vi "DSC TSV PRE-Process Files with Queues.vi"() -> ()   [LabVIEW 2019, in "LV-Data.PGSQL.lvclass"]
uses:
  LV-Data.PGSQL.lvclass
  <userlib>/_OpenG.lib/file/file.llb/Build Path - File Names Array__ogtk.vi
panel:
  out "appended path":path
  out "read loop":i32
  in  "Stop":bool
  out "conversion loop":i32
  in  "Folders":path
  in  "Number of row to read \nat a time":i32=10000
  in  "error in":errorcluster
  out "error out":errorcluster
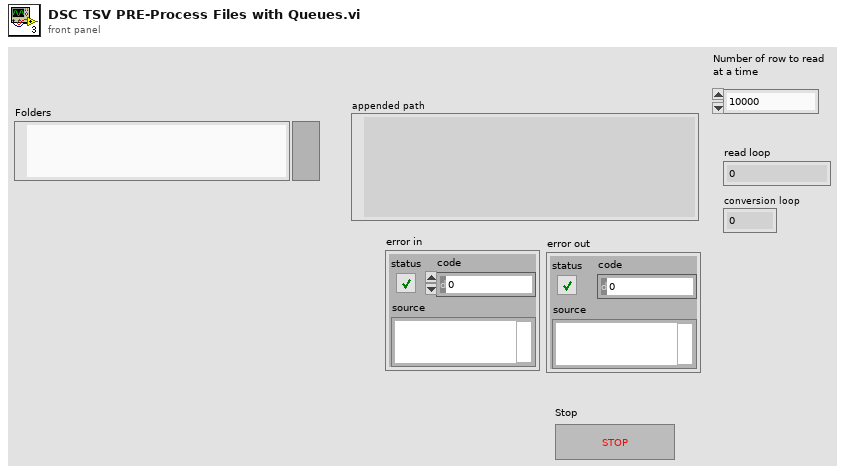
[diagram p1: front panel]
types:
  T1 = enum16{"open", "replace", "create", "open or create", "replace or create", "replace or create with confirmation"}
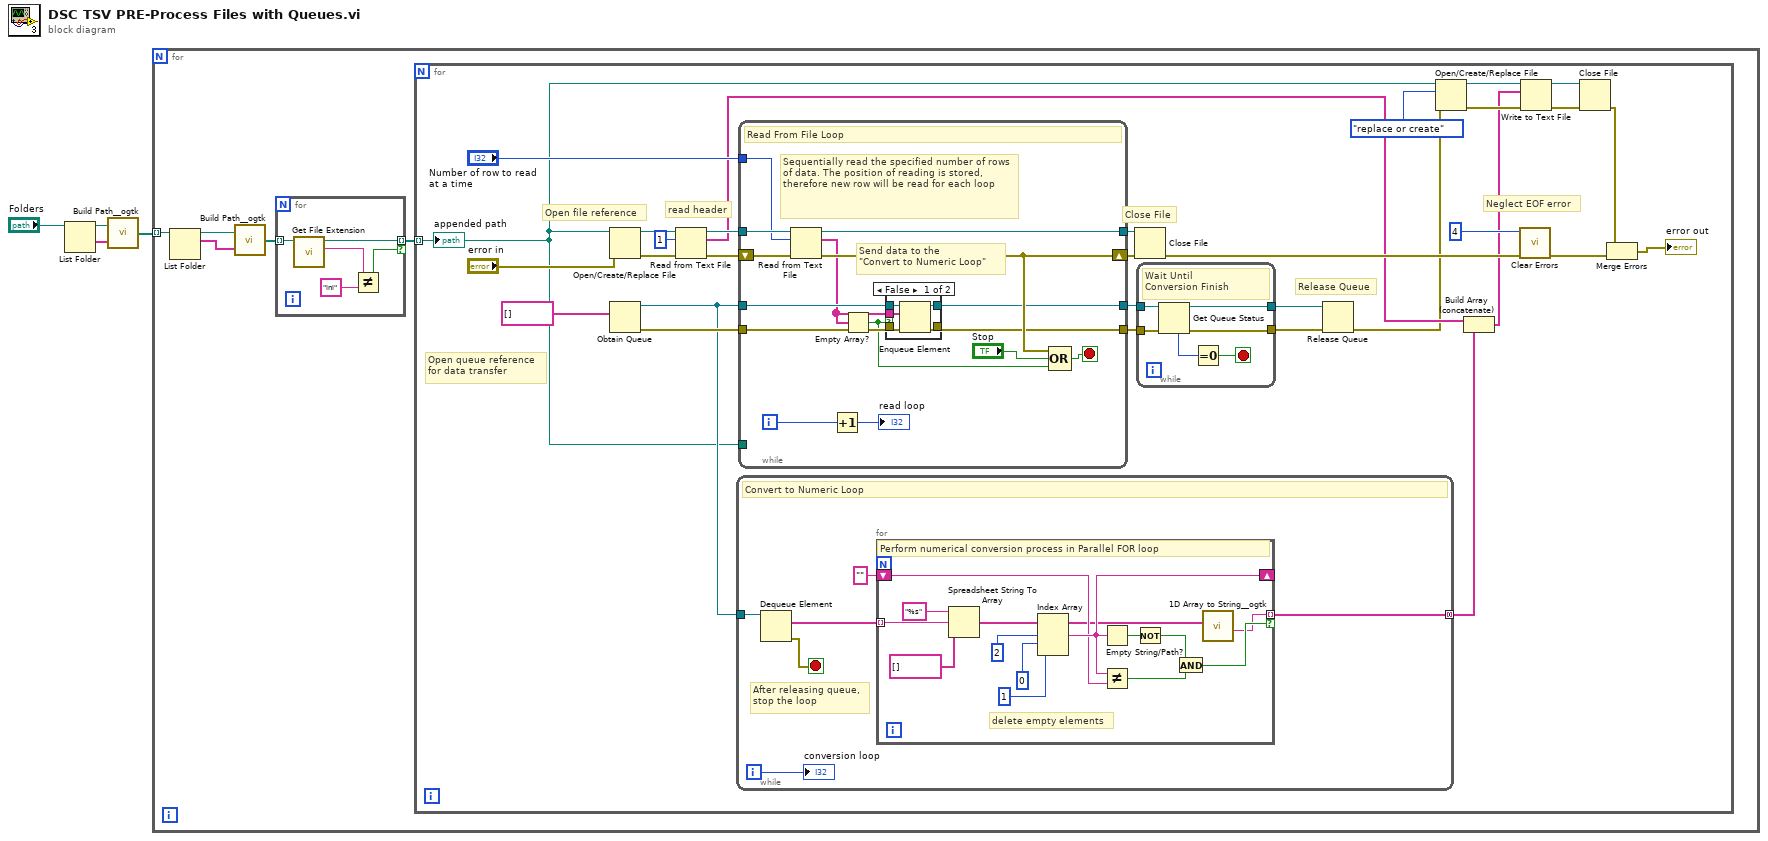
[diagram p0: block diagram]
diagram:
  n1 = List Folder(path="Folders") -> (path out=w3:path, folder names=w4:string[])  [unwired: 3 in, 2 out]
  n2 = call-poly <userlib>:"Build Path__ogtk.vi"("name or relative path"=w4, "base path"=w3) -> ("appended path"=w2:path[])
  n3 = for {
    tunnel: w2 -> [w9] mode=indexing
    n4 = List Folder(path=w9) -> (path out=w8:path, filenames=w7:string[])  [unwired: 3 in, 2 out]
    n5 = call-poly <userlib>:"Build Path__ogtk.vi"("name or relative path"=w7, "base path"=w8) -> ("appended path"=w6:path[])
    n6 = for {
      tunnel: w6 -> [w14] mode=indexing
      tunnel: [w13] -> w5 mode=indexing if=w10
      n7 = call <vilib>:"Get File Extension.vi"("file"=w14) -> ("lowercase file extension"=w12:string, "dup file"=w13:path)  [unwired: 6 in, 3 out]
      n8 = Not Equal?(x=w12, y="ini") -> (x != y?=w10:bool)
    }
    n9 = for {
      tunnel: w5 -> [w17] mode=indexing
      # "read header"
      # "Neglect EOF error"
      # "Release Queue"
      # "Close File"
      # "Open queue reference\nfor data transfer"
      # "Open file reference"
      n10 = Open/Create/Replace File(file path (use dialog)=w17, error in="error in") -> (refnum out=w34:refnum<file>, error out=w31:errorcluster)  [unwired: 4 in, 1 out]
      n11 = Obtain Queue(element data type=string[] [] ("形式文字列")) -> (queue out=w39:refnum<queue>, error out=w40:errorcluster)  [unwired: 4 in, 1 out]
      n12 = Read from Text File(file (use dialog)=w34, count=1, error in=w31) -> (refnum out=w33:refnum<file>, text=w23:string[], error out=w32:errorcluster)  [unwired: 1 in, 1 out]
      n13 = while {
        tunnel: w39 -> [w51]
        tunnel: [w46] -> w25 mode=concatenating
        i -> [w49]
        stop <- w50 stop-if-true
        # "After releasing queue,\nstop the loop"
        # "Convert to Numeric Loop"
        n14 = Dequeue Element(queue=w51) -> (element=w48:string[], error out=w50:errorcluster)  [unwired: 2 in, 2 out]
        n15 = for "Forループ" {
          tunnel: w48 -> [w63] mode=indexing
          tunnel: [w52] -> w46 mode=indexing if=w54
          shift-right: [w58] -> _
          shift-left: "" ("String") -> [w57]
          # "delete empty elements"
          # "Perform numerical conversion process in Parallel FOR loop"
          n16 = Spreadsheet String To Array(format string="%s", spreadsheet string=w63, array type (2D Dbl)=string[] []) -> (array=w53:string[])  [unwired: 1 in]
          n17 = Index Array(array=w53, index #1=2 ("disabled index (col)"), index #2=0 ("disabled index (col)"), index #3=1 ("disabled index (col)")) -> (element #1=w58:string)  [unwired: 2 out]
          n18 = Empty String/Path?(string/path=w58) -> (empty?=w59:bool)
          n19 = Not Equal?(x=w58, y=w57) -> (x != y?=w55:bool)
          n20 = Not(x=w59) -> (.not. x?=w56:bool)
          n21 = And(x=w56, y=w55) -> (x .and. y?=w54:bool)
          n22 = call <userlib>:"1D Array to String__ogtk.vi"("Array of Strings"=w53) -> ("delimited string"=w52:string)  [unwired: 10 in]
        }
        "conversion loop" <- w49
      }
      n23 = while {
        tunnel: w33 -> [w80]
        tunnel: [w78] -> w45
        shift-right: [w74] -> w44
        shift-left: w32 -> [w79]
        tunnel: "Number of row to read \nat a time" -> [w75]
        tunnel: w39 -> [w73]
        tunnel: w40 -> [w72]
        tunnel: [w71] -> w38
        tunnel: [w70] -> w37
        tunnel: w17 -> [_]
        i -> [w76]
        stop <- w77 stop-if-true
        # "Send data to the \n\"Convert to Numeric Loop\""
        # "Sequentially read the specified number of rows of data. The position of reading is stored, therefore new row will be read for each loop"
        # "Read From File Loop"
        n24 = Read from Text File(file (use dialog)=w80, count=w75, error in=w79) -> (refnum out=w78:refnum<file>, text=w68:string[], error out=w74:errorcluster)  [unwired: 1 in, 1 out]
        n25 = Increment(x=w76) -> (x+1=→"read loop":i32)
        n26 = Empty Array?(array=w68) -> (empty?=w66:bool)
        n27 = case shown="False" w66 {
          tunnel: w73 -> [w85 w87]
          tunnel: w72 -> [w84 w86]
          tunnel: [w83 w87] -> w71
          tunnel: [w82 w86] -> w70
          tunnel: w68 -> [w81 _]
          frame False {
            n28 = Enqueue Element(queue=w85, element=w81, error in (no error)=w84) -> (queue out=w83:refnum<queue>, error out=w82:errorcluster)  [unwired: 1 in, 1 out]
          }
          frame True {
          }
        }
        n29 = Compound Arithmetic op=OR(w74, "Stop", w66) -> (w77:bool)
      }
      n30 = Close File(refnum=w45, error in=w44) -> (error out=w43:errorcluster)  [unwired: 1 out]
      n31 = while {
        tunnel: w38 -> [w93]
        tunnel: w37 -> [w92]
        tunnel: [w89] -> w35
        tunnel: [w88] -> w36
        stop <- w90 stop-if-true
        # "Wait Until \nConversion Finish"
        n32 = Get Queue Status(queue=w93, error in (no error)=w92) -> (queue out=w89:refnum<queue>, error out=w88:errorcluster, # elements in queue=w91:i32)  [unwired: 1 in, 5 out]
        n33 = Equal To 0?(x=w91) -> (x = 0?=w90:bool)
      }
      n34 = Release Queue(queue=w35, error in (no error)=w36) -> (error out=w18:errorcluster)  [unwired: 1 in, 2 out]
      n35 = Open/Create/Replace File(file path (use dialog)=w17, error in=w18, operation (0:open)=T1."replace or create") -> (refnum out=w21:refnum<file>, error out=w24:errorcluster)  [unwired: 3 in, 1 out]
      n36 = Build Array (concatenate)(w23, w25) -> (w22:string[])
      n37 = call <vilib>:"Clear Errors.vi"("error in (no error)"=w43, "specific error code to clear (0: all)"=4) -> ("error out"=w16:errorcluster)  [unwired: 4 in, 1 out]
      n38 = Write to Text File(file (use dialog)=w21, text=w22, error in=w24) -> (refnum out=w19:refnum<file>, error out=w20:errorcluster)  [unwired: 1 in, 1 out]
      n39 = Close File(refnum=w19, error in=w20) -> (error out=w15:errorcluster)  [unwired: 1 out]
      n40 = Merge Errors(w15, w16) -> (→"error out":errorcluster)
      "appended path" <- w17
    }
  }
